vi "NEW_PRN Generation_Station2.vi"(8 "error in (no error)":errorcluster, 11 "ClusterIN":T2) -> (0 "error out":errorcluster, 1 "ClusterOUT":T2, 3 "QR CODE":string)   [LabVIEW 2017]
uses:
  <vilib>/addons/database/Connection.llb/Conn ObjectReference.ctl
  <vilib>/addons/database/NI_Database_API.lvlib
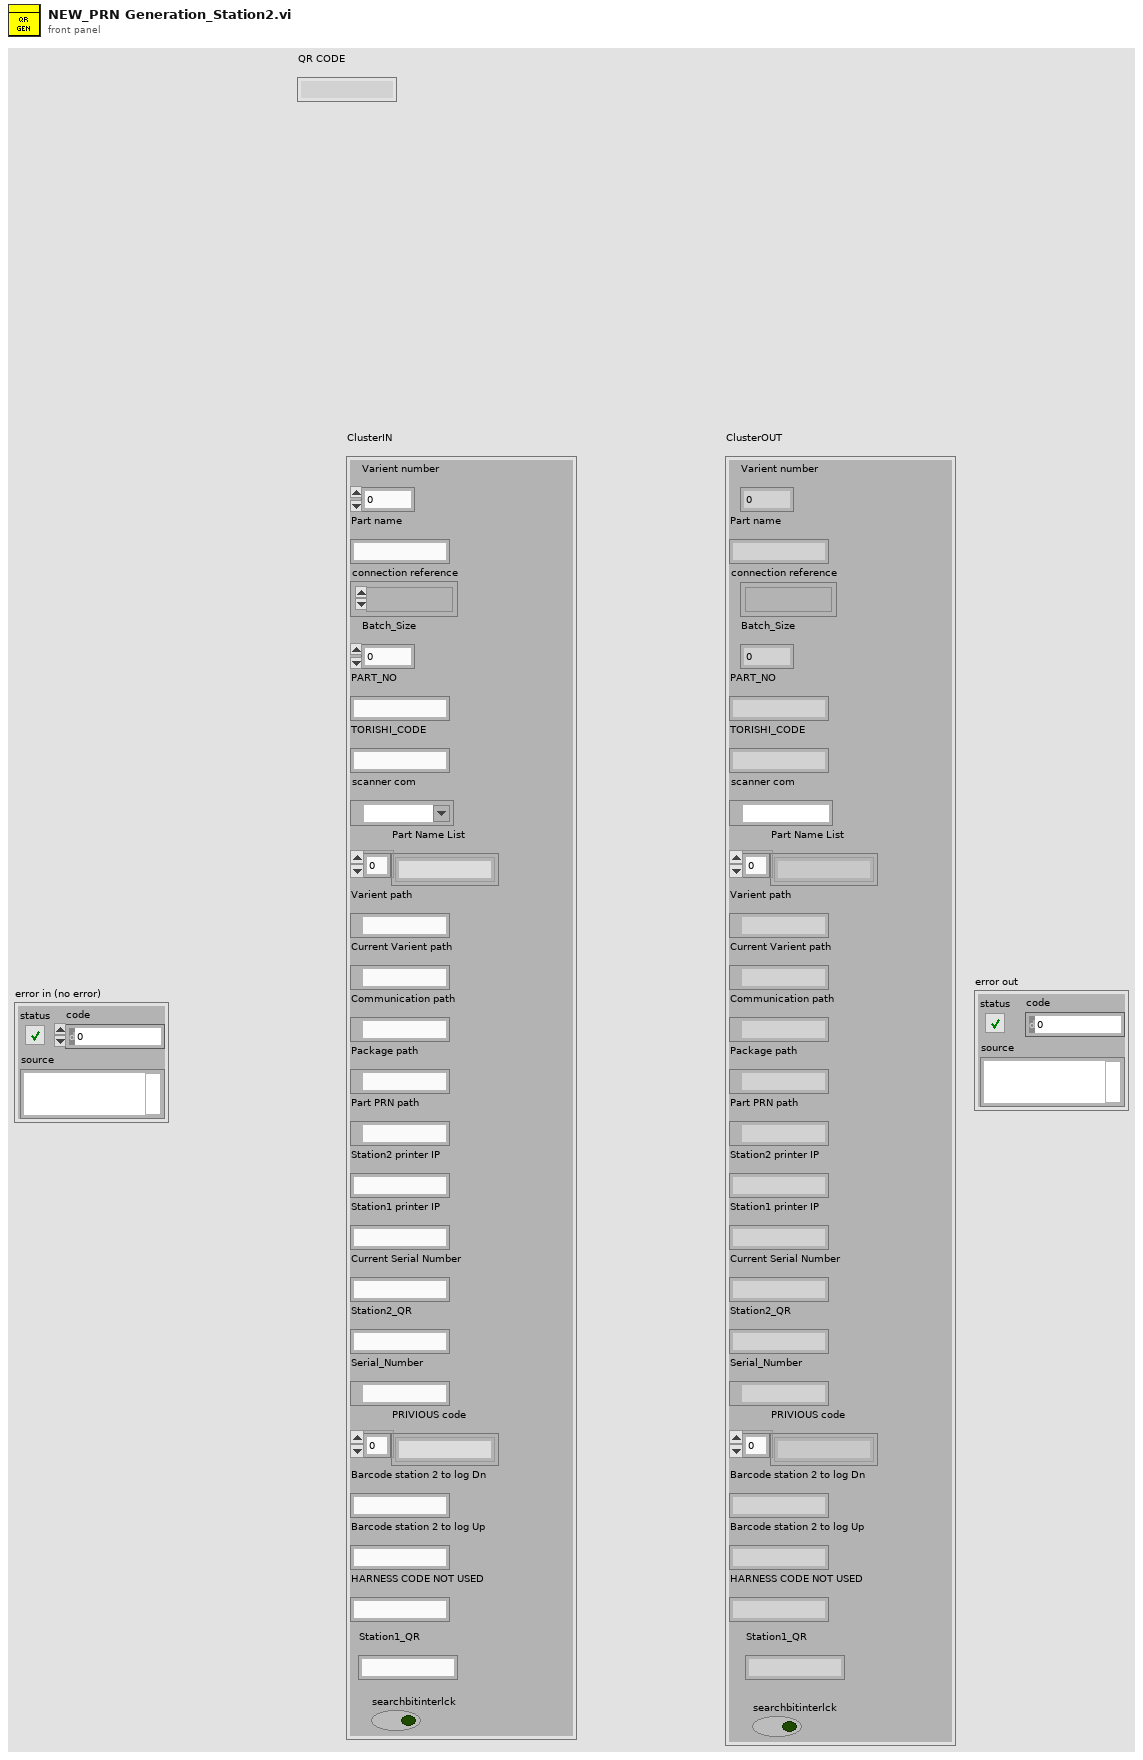
[diagram p1: front panel]
types:
  T1 = typedef "NI_Database_API.lvlib/Conn ObjectReference.ctl" = refnum<k1>
  T2 = cluster{"Varient number":u16, "Part name":string, "connection reference":T1, "Batch_Size":u16, "PART_NO":string, "TORISHI_CODE":string, "scanner com":refnum<visa-resource-name>, "Part Name List":string[], "Varient path":path, "Current Varient path":path, "Communication path":path, "Package path":path, "Part PRN path":path, "Station2 printer IP":string, "Station1 printer IP":string, "Current Serial Number":string, "Station2_QR":string, "Serial_Number":path, "PRIVIOUS code":string[], "Barcode station 2 to log Dn":string, "Barcode station 2 to log Up":string, "HARNESS CODE NOT USED":string, "Station1_QR":string, "searchbitinterlck":bool}
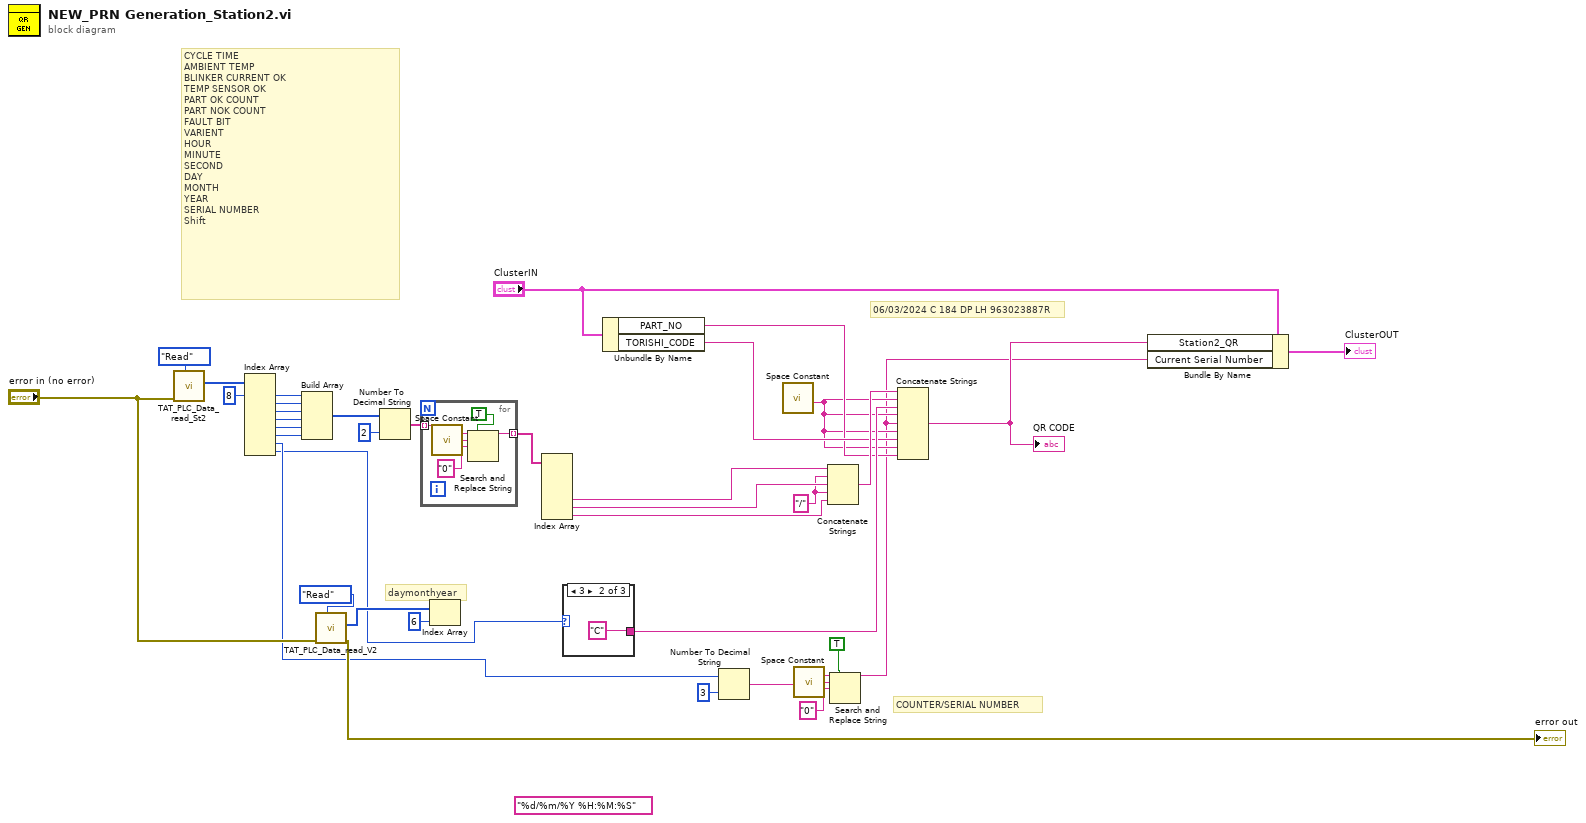
[diagram p0: block diagram]
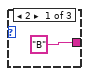
[diagram p2: hidden frame]
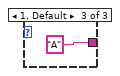
[diagram p3: hidden frame]
diagram:
  w4 = "/"
  (unwired) "%d/%m/%Y %H:%M:%S" ("time format string (%c)")
  # "06/03/2024 C 184 DP LH 963023887R"
  # "CYCLE TIME\nAMBIENT TEMP\nBLINKER CURRENT OK\nTEMP SENSOR OK\nPART OK COUNT\nPART NOK COUNT\nFAULT BIT\nVARIENT\nHOUR\nMINUTE\nSECOND\nDAY\nMONTH\nYEAR\nSERIAL NUMBER\nShift"
  # "COUNTER/SERIAL NUMBER"
  # "daymonthyear"
  n1 = call "TAT_PLC_Data_read_St2.vi"("Enum"=enum16{"Read", "Write"}."Read", "error in (no error)"="error in (no error)") -> ("Array 2"=w27:u16[])  [unwired: 8 in, 1 out]
  n2 = Index Array(array=w27, index #1=8 ("index")) -> (element #1=w24:u16, element #2=w23:u16, element #3=w22:u16, element #4=w21:u16, element #5=w20:u16, element #6=w19:u16, element #7=w16:u16, element #8=w3:u16)  [unwired: 7 in]
  n3 = Build Array(w24, w23, w22, w21, w20, w19) -> (w17:u16[])
  n4 = call "TAT_PLC_Data_read_V2.vi"("Enum"=enum16{"Read", "Write"}."Read", "error in (no error)"="error in (no error)") -> ("error out"=→"error out":errorcluster, "Array 2"=w18:u16[])  [unwired: 8 in]
  n5 = Number To Decimal String(number=w17, width (-)=i16 2) -> (decimal integer string=w30:string[])
  n6 = for {
    tunnel: w30 -> [w40] mode=indexing
    tunnel: [w39] -> w29 mode=indexing
    n7 = call <vilib>:"Space Constant.vi"() -> ("String"=w41:string)
    n8 = Search and Replace String(replace all?=TRUE ("replace all? (F)"), input string=w40, search string=w41, replace string="0" ("replace string (\"\")")) -> (result string=w39:string)  [unwired: 4 in, 3 out]
  }
  n9 = Index Array(array=w18, index=6) -> ()  [unwired: 1 out]
  n10 = Index Array(array=w29) -> (element #4=w6:string, element #5=w15:string, element #6=w5:string)  [unwired: 6 in, 3 out]
  n11 = case shown="3" w3 {
    tunnel: ["B" "C" "A"] -> w11
    frame 2 {
    }
    frame 3 {
    }
    frame 1, Default {
    }
  }
  n12 = Unbundle By Name("ClusterIN") -> ("PART_NO"=w9:string, "TORISHI_CODE"=w10:string)
  n13 = Number To Decimal String(number=w16, width (-)=i16 3) -> (decimal integer string=w2:string)
  n14 = call <vilib>:"Space Constant.vi"() -> ("String"=w7:string)
  n15 = call <vilib>:"Space Constant.vi"() -> ("String"=w33:string)
  n16 = Concatenate Strings(w6, w4, w15, w4, w5) -> (w12:string)
  n17 = Search and Replace String(replace all?=TRUE ("replace all? (F)"), input string=w2, search string=w33, replace string="0" ("replace string (\"\")")) -> (result string=w1:string)  [unwired: 4 in, 3 out]
  n18 = Concatenate Strings(w12, w7, w11, w7, w1, w7, w10, w7, w9) -> (w8:string)
  "QR CODE" <- w8
  n19 = Bundle By Name(cluster="ClusterIN", "Station2_QR"=w8, "Current Serial Number"=w1) -> (→"ClusterOUT":T2)
